vi "Flow Rate Register Data to Value Unit.vi"(0 "Value Reg Data":u16=1 caption="数值寄存器", 3 "Unit Reg Data":u16=100 caption="单位寄存器") -> (7 "Flow Rate Value":dbl=100.0 caption="流量值", 10 "Flow Rate Unit":string caption="流量单位")   [LabVIEW 2023, in "Longer Pump dLSP501 Series.lvlib"]
uses:
  <instrlib>/Longer Pump dLSP501 Modbus RTU Series/Longer Pump dLSP501 Series.lvlib
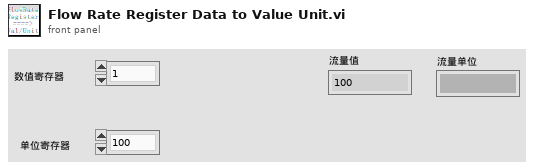
[diagram p1: front panel]
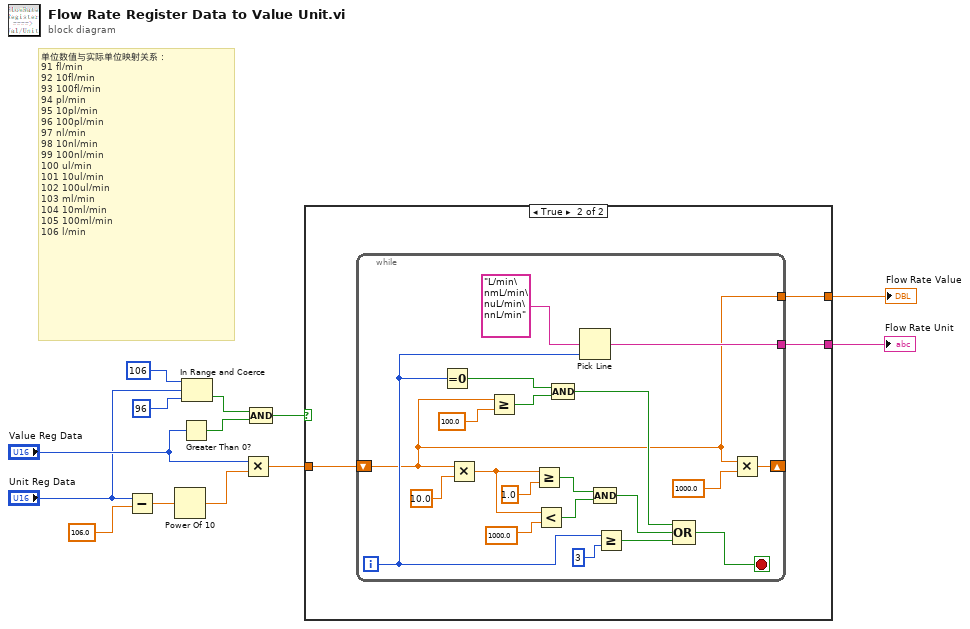
[diagram p0: block diagram]
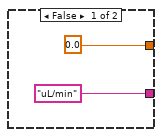
[diagram p2: hidden frame]
diagram:
  # "单位数值与实际单位映射关系：\n91\tfl/min\n92\t10fl/min\n93\t100fl/min\n94\tpl/min\n95\t10pl/min\n96\t100pl/min\n97\tnl/min\n98\t10nl/min\n99\t100nl/min\n100\tul/min\n101\t10ul/min\n102\t100ul/min\n103\tml/min\n104\t10ml/min\n105\t100ml/min\n106\tl/min"
  n1 = Subtract(x="Unit Reg Data", y=106.0) -> (x-y=w12:dbl)
  n2 = Power Of 10(x=w12) -> (10^x=w11:dbl)
  n3 = Greater Than 0?(x="Value Reg Data") -> (x > 0?=w5:bool)
  n4 = In Range and Coerce(upper limit=u16 106 ("上限"), x="Unit Reg Data", lower limit=u16 96 ("下限")) -> (In Range?=w4:bool)  [unwired: 1 out]
  n5 = Multiply(x="Value Reg Data", y=w11) -> (x*y=w9:dbl)
  n6 = Compound Arithmetic op=AND ("复合运算")(w4, w5) -> (w3:bool)
  n7 = case shown="True" w3 {
    tunnel: w9 -> [_ w18]
    tunnel: ["uL/min" w17] -> w8
    tunnel: [0.0 ("x") w16] -> w7
    frame False {
    }
    frame True {
      n8 = while {
        tunnel: [w27] -> w17
        tunnel: [w19] -> w16
        shift-right: [w26] -> _
        shift-left: w18 -> [w19]
        i -> [w25]
        stop <- w29 stop-if-true
        n9 = Equal To 0?(x=w25) -> (x = 0?=w23:bool)
        n10 = Multiply(x=w19, y=10.0 ("y 2")) -> (x*y=w36:dbl)
        n11 = Greater Or Equal?(x=w19, y=100.0 ("y 2")) -> (x >= y?=w22:bool)
        n12 = Greater Or Equal?(x=w36, y=1.0) -> (x >= y?=w34:bool)
        n13 = Less?(x=w36, y=1000.0) -> (x < y?=w33:bool)
        n14 = Compound Arithmetic op=AND ("复合运算")(w23, w22) -> (w21:bool)
        n15 = Pick Line(multi-line string="L/min\nmL/min\nuL/min\nnL/min", line index=w25) -> (output string=w27:string)  [unwired: 1 in]
        n16 = Compound Arithmetic op=AND ("复合运算")(w34, w33) -> (w30:bool)
        n17 = Greater Or Equal?(x=w25, y=3) -> (x >= y?=w31:bool)
        n18 = Compound Arithmetic op=OR ("复合运算")(w21, w30, w31) -> (w29:bool)
        n19 = Multiply(x=w19, y=1000.0 ("y 2")) -> (x*y=w26:dbl)
      }
    }
  }
  "Flow Rate Value" <- w7
  "Flow Rate Unit" <- w8
